vi "const_cluster_svcan3settings.vi"() -> (0 "SVCAN3Settings":T1)   [LabVIEW 2009]
doc: "this vi returns the SVCAN3setting cluster\n\n12/22/2010 1.0.0 jyg\n- initial release"
uses:
  ctl svcansetting.ctl
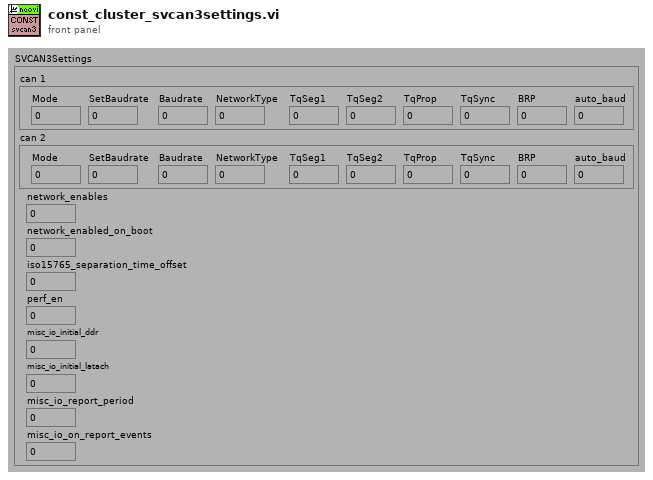
[diagram p1: front panel]
types:
  T1 = typedef "ctl SVCANSetting.ctl" = cluster{"can 1":cluster{"Mode":u8, "SetBaudrate":u8, "Baudrate":u8, "NetworkType":u8, "TqSeg1":u8, "TqSeg2":u8, "TqProp":u8, "TqSync":u8, "BRP":u16, "auto_baud":u16}, "can 2":cluster{"Mode":u8, "SetBaudrate":u8, "Baudrate":u8, "NetworkType":u8, "TqSeg1":u8, "TqSeg2":u8, "TqProp":u8, "TqSync":u8, "BRP":u16, "auto_baud":u16}, "network_enables":u16, "network_enabled_on_boot":u16, "iso15765_separation_time_offset":i16, "perf_en":u16, "misc_io_initial_ddr":u16, "misc_io_initial_latach":u16, "misc_io_report_period":u16, "misc_io_on_report_events":u16}
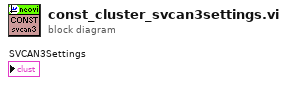
[diagram p0: block diagram]
diagram:
